vi "UHR-Fleezers Control (host) - 11.1.vi"() -> ()   [LabVIEW 2012] (continued)
                n290 = Multiply(x=w512, y=w521) -> (x*y=w531:dbl)
                n291 = Divide "X half step offset"(x=w509, y=2.0) -> (x/y=w517:dbl)
                n292 = Divide "X V/pix"(x=w509, y=w520) -> (x/y=w519:dbl)
                n293 = Multiply(x=w509, y=w514) -> (x*y=w526:dbl)
                n294 = Compound Arithmetic op=ADD(w524, w531, w530) -> (w501:dbl)
                "Pointer Y (V)" <- w501
                n295 = Multiply(x=w519, y=w513) -> (x*y=w528:dbl)
                n296 = Negate(x=w517) -> (-x=w516:dbl)
                n297 = local read "Initial X"() -> (w529:dbl)
                n298 = Negate(x=w528) -> (-x=w527:dbl)
                n299 = Compound Arithmetic op=ADD(w516, w526, w529, w527) -> (w502:dbl)
                "Pointer X (V)" <- w502
                n300 = case shown="True" "Set High F Confocal Spot (X-Y)" {
                  tunnel: w502 -> [_ w532]
                  tunnel: w501 -> [_ w533]
                  frame False {
                  }
                  frame True {
                    "Confocal Y 2 (V)" <- w533
                    "Confocal X 2 (V)" <- w532
                  }
                }
                n301 = Or(x="Set X Only", y="Set Confocal Spot (X-Y)") -> (x .or. y?=w505:bool)
                n302 = Or(x="Set Confocal Spot (X-Y)", y="Set Y Only") -> (x .or. y?=w504:bool)
                n303 = case shown="True" w505 {
                  tunnel: w502 -> [_ w534]
                  frame False {
                  }
                  frame True {
                    n304 = property on="AO2" class="Slide (strict)"("Val(Sgnl)"=w534) -> ()  [unwired: 2 in, 2 out]
                    "Confocal X 1 (V)" <- w534
                  }
                }
                n305 = case shown="True" w504 {
                  tunnel: w501 -> [_ w535]
                  frame False {
                  }
                  frame True {
                    n306 = property on="AO1" class="Slide (strict)"("Val(Sgnl)"=w535) -> ()  [unwired: 2 in, 2 out]
                    "Confocal Y 1 (V)" <- w535
                  }
                }
                n307 = local write "Set High F Confocal Spot (X-Y)"(w500) -> ()
                n308 = local write "Set Confocal Spot (X-Y)"(w500) -> ()
                n309 = local write "Set X Only"(w500) -> ()
                n310 = local write "Set Y Only"(w500) -> ()
              }
            }
          }
          frame 3 {
            n311 = local read "BD 2 Frequency 1 (MHz)"() -> (w536:dbl)
            n312 = local read "BD 1 Frequency 1 (MHz)"() -> (w537:dbl)
            n313 = local write "Manipulating Trap"(TRUE ("Manipulating Trap")) -> ()
            n314 = local write "Coords"(T7 {"Horizontal"=0, "Vertical"=0} ("Coords")) -> ()
            n315 = while {
              tunnel: w542 -> [w547]
              tunnel: w540 -> [w546]
              tunnel: w538 -> [w545]
              tunnel: w537 -> [w544]
              tunnel: w536 -> [w543]
              stop <- w548 stop-if-true
              n316 = event shown="[0] \"Pane\": Mouse Move" {
                selector: _ -> [_ _]
                dyn-events: _ -> [_ _]
                timeout: _ -> [_ _]
                tunnel: ["Force Manip Abort" w612] -> w548
                tunnel: w547 -> [w555 _]
                tunnel: w546 -> [w553 _]
                tunnel: w545 -> [w552 _]
                tunnel: w544 -> [w551 _]
                tunnel: w543 -> [w550 _]
                event Mouse Move {
                  n317 = event-data() -> ("Time"=w556:u32, "Coords"=w557:T7)  [unwired: 3 out]
                  n318 = Less?(x=w556, y=w555) -> (x < y?=w554:bool)
                  n319 = case "Makes sure old motion events prior to mouse click aren't used" shown="False" w554 {
                    tunnel: w557 -> [w599 _]
                    tunnel: w553 -> [w600 _]
                    tunnel: w552 -> [w577 _]
                    tunnel: w551 -> [w573 _]
                    tunnel: w550 -> [w572 _]
                    frame False {
                      n320 = Subtract(x=w599, y=w600) -> (x-y=w598:T7)
                      "Coords" <- w598
                      n321 = local read "Y RF Frequency Limits (MHz)"() -> (w558:T16)
                      n322 = To Double Precision Float(number=w598) -> (double precision float=w597:cluster{"Horizontal":dbl, "Vertical":dbl})
                      n323 = Multiply(x=cluster{"Horizontal":dbl, "Vertical":dbl} {"Horizontal"=-1.0, "Vertical"=1.0}, y="Manipulation Scaling") -> (x*y=w593:cluster{"Horizontal":dbl, "Vertical":dbl})
                      n324 = local read "X RF Frequency Limits (MHz)"() -> (w559:T16)
                      n325 = Multiply(x=w597, y=w593) -> (x*y=w595:cluster{"Horizontal":dbl, "Vertical":dbl})
                      n326 = Unbundle By Name(w595) -> ("Horizontal"=w590:dbl, "Vertical"=w594:dbl)
                      n327 = Unbundle By Name(w558) -> ("Maximum"=w561:dbl, "Minimum"=w560:dbl)
                      n328 = Boolean To (0,1)(Boolean="Manip. X?") -> (0, 1=w588:i16)
                      n329 = Boolean To (0,1)(Boolean="Manip. Y?") -> (0, 1=w585:i16)
                      n330 = local read "BD 1 Frequency 2 (MHz)"() -> (w575:dbl)
                      n331 = Multiply(x=w594, y=w585) -> (x*y=w587:dbl)
                      n332 = Multiply(x=w588, y=w590) -> (x*y=w591:dbl)
                      n333 = local read "BD 2 Frequency 2 (MHz)"() -> (w574:dbl)
                      n334 = Unbundle By Name(w559) -> ("Maximum"=w563:dbl, "Minimum"=w562:dbl)
                      n335 = Add(x=w572, y=w587) -> (x+y=w565:dbl)
                      n336 = Add(x=w573, y=w591) -> (x+y=w567:dbl)
                      n337 = In Range and Coerce(upper limit=w563, x=w567, lower limit=w562) -> (coerced(x)=w566:dbl)  [unwired: 1 out]
                      n338 = In Range and Coerce(upper limit=w561, x=w565, lower limit=w560) -> (coerced(x)=w564:dbl)  [unwired: 1 out]
                      n339 = Subtract(x=w566, y=w575) -> (x-y=w584:dbl)
                      n340 = Subtract(x=w564, y=w574) -> (x-y=w583:dbl)
                      n341 = Square(x=w584) -> (x^2=w582:dbl)
                      n342 = Square(x=w583) -> (x^2=w581:dbl)
                      n343 = Add(x=w582, y=w581) -> (x+y=w580:dbl)
                      n344 = Square Root(x=w580) -> (sqrt(x)=w576:dbl)
                      n345 = In Range and Coerce(upper limit="Limit Max (MHz)", x=w576, lower limit="Limit Min (MHz)") -> (In Range?=w569:bool)  [unwired: 1 out]
                      n346 = Not(x="Limits Enable") -> (.not. x?=w568:bool)
                      n347 = Or(x=w569, y=w568) -> (x .or. y?=w570:bool)
                      n348 = case shown="True" w570 {
                        tunnel: w577 -> [_ w610]
                        tunnel: w576 -> [_ w601]
                        tunnel: w566 -> [_ w608]
                        tunnel: w575 -> [_ w607]
                        tunnel: w564 -> [_ w606]
                        tunnel: w574 -> [_ w605]
                        tunnel: w559 -> [_ w603]
                        tunnel: w558 -> [_ w602]
                        frame False {
                        }
                        frame True {
                          n349 = local read "BD 1 Frequency 3 (MHz)"() -> (w609:dbl)
                          n350 = local read "BD 2 Frequency 3 (MHz)"() -> (w604:dbl)
                          n351 = local write "Trap Delta (MHz)"(w601) -> ()
                          n352 = call "set RF board frequency - interlace.vi"("Board 2 Frequency Limits"=w602, "Board 1 Frequency Limits"=w603, "FPGA VI Reference In"=w610, "Board 2 Frequency 3 (MHz)"=w604, "Board 1 Frequency 3 (MHz)"=w609, "Board 2 Frequency 2 (MHz)"=w605, "Board 2 Frequency 1 (MHz)"=w606, "Board 1 Frequency 2 (MHz)"=w607, "Board 1 Frequency 1  (MHz)"=w608) -> ()  [unwired: 1 in, 2 out]
                          n353 = local write "BD 2 Frequency 1 (MHz)"(w606) -> ()
                          n354 = local write "BD 1 Frequency 1 (MHz)"(w608) -> ()
                        }
                      }
                    }
                    frame True {
                    }
                  }
                }
                event Mouse Up {
                  n355 = event-data() -> ("Button"=w611:u16)  [unwired: 8 out]
                  n356 = case shown="3" w611 {
                    tunnel: [FALSE TRUE] -> w612
                    frame 0, Default {
                    }
                    frame 3 {
                      n357 = local read "Trap Delta (MHz)"() -> (w614:dbl)
                      n358 = property on="Initial delta (MHz)" class="DigNum (strict)"("Val(Sgnl)"=w614) -> ()  [unwired: 2 in, 2 out]
                      n359 = local write "Manipulating Trap"(FALSE ("Manipulating Trap")) -> ()
                    }
                  }
                }
              }
            }
          }
        }
      }
      event Mouse Move {
        n360 = event-data() -> ()  [unwired: 6 out]
      }
    }
    n361 = local read "Stop All"() -> (w430:bool)
    n362 = node-c288() -> ()  [unwired: 2 out]
  }
  n363 = timed-loop "Run Scripts, including: stage motion" {
    tunnel: w89 -> [w623]
    tunnel: w88 -> [w624]
    tunnel: [w624] -> w87
    tunnel: [w623] -> w86
    timing: w84 -> [_]
    timing-out: [_] -> w83
    tunnel: w69 -> [w622]
    tunnel: w70 -> [w621]
    tunnel: w10 -> [w618]
    tunnel: w9 -> [w617]
    tunnel: w8 -> [w619]
    tunnel: w7 -> [w620]
    stop <- w625 stop-if-true
    n364 = node-c288() -> ()  [unwired: 1 in, 1 out]
    n365 = event shown="[3] \"Move Cap. 2 (ADig Top)\": Value Change" {
      selector: _ -> [_ _ _ _ _ _ _ _ _ _ _ _ _ _ _ _ _ _ _]
      dyn-events: _ -> [_ _ _ _ _ _ _ _ _ _ _ _ _ _ _ _ _ _ _]
      timeout: _ -> [_ _ _ _ _ _ _ _ _ _ _ _ _ _ _ _ _ _ _]
      tunnel: ["Set Position" "Move to Position" _ _ "Read Harvard" _ _ _ _ _ _ "Got ADig bead" "Force FB Data\nScript" _ "Got DNA bead" "Take Stepping Data" _ "Take Detection Laser\nImage" _] -> _
      tunnel: [_ _ _ _ _ _ _ _ _ _ _ _ _ _ _ _ _ _ w1242] -> w625
      tunnel: w623 -> [w643 w651 w664 w694 _ w739 w779 w860 w889 w1021 w1047 _ w1083 _ _ _ _ _ _]
      tunnel: w624 -> [w644 w652 w665 w695 _ w740 w780 w861 w890 w1022 w1048 _ w1084 _ _ _ _ _ _]
      tunnel: w622 -> [_ _ _ _ w724 _ _ _ _ _ _ _ _ _ _ _ _ _ _]
      tunnel: w621 -> [_ _ _ _ w723 _ _ _ _ _ _ _ _ _ _ _ _ _ _]
      tunnel: w620 -> [_ _ _ _ _ _ _ _ _ _ _ _ _ _ _ _ _ _ _]
      tunnel: w619 -> [_ _ _ _ _ _ _ _ _ _ _ _ _ _ _ _ _ _ _]
      tunnel: w618 -> [_ _ _ _ _ _ _ _ _ _ _ _ _ _ _ _ _ _ _]
      tunnel: w617 -> [_ _ _ _ _ _ _ _ _ _ _ _ _ _ _ _ _ _ _]
      event "Set Position", "Set Position 2", "Set Position 3", "Set Position 4", "Set Position 5", "Set Position 1": Value Change {
        n366 = event-data() -> ()  [unwired: 1 in, 5 out]
        n367 = Build Array("Set Position 1", "Set Position 2", "Set Position 3", "Set Position 4", "Set Position 5") -> (w642:bool[])
        n368 = Boolean Array To Number(Boolean array=w642) -> (number=w641:u32)
        n369 = Logarithm Base 2(1:w641) -> (0:w633:dbl)
        n370 = call "Read Stage Position.vi"("error in"=w643, "VISA resource name in"=w644) -> ("Current Position"=w648:cluster{dbl, dbl, dbl}, "error out"=w647:errorcluster)  [unwired: 2 out]
        n371 = Decrement(x="Position") -> (x-1=w631:dbl)
        n372 = Greater Or Equal?(x=w633, y=0.0) -> (x >= y?=w634:bool)
        n373 = Cluster To Array(cluster=w648) -> (array=w645:dbl[])
        n374 = local write "Stage Control Serial Error"(w647) -> ()
        n375 = Select(t=w633, s=w634, f=w631) -> (s? t:f=w630:dbl)
        n376 = Increment(x=w630) -> (x+1=w629:dbl)
        n377 = Build Array (concatenate)(w629, w645) -> (w628:dbl[])
        n378 = Replace Array Subset(array="Saved Stage Positions", new element=w628, index (row)=w630) -> (w646:dbl[][])  [unwired: 1 in]
        n379 = local write "Saved Stage Positions"(w646) -> ()
      }
      event "Move to Position": Value Change {
        n380 = event-data() -> ()  [unwired: 1 in, 5 out]
        n381 = flat-sequence {
          tunnel: w652 -> [w656]
          tunnel: w651 -> [w655]
          frame #0 {
            n382 = local read "Saved Stage Positions"() -> (w658:dbl[][])
            n383 = local read "Position"() -> (w657:dbl)
            n384 = local write "Stage Moving"(TRUE ("Stage Moving")) -> ()
            n385 = call "move to saved stage position.vi"("error in"=w655, "Stage VISA resource name in"=w656, "Position"=w657, "Saved Stage Positions"=w658) -> ("error out"=w654:errorcluster)  [unwired: 1 out]
            n386 = local write "Stage Control Serial Error"(w654) -> ()
          }
          frame #1 {
            n387 = call <vilib>:"Beep.vi"() -> ()  [unwired: 3 in, 9 out]
            n388 = local write "Stage Moving"(FALSE ("Stage Moving")) -> ()
          }
        }
      }
      event "Move Cap. 1 (DNA Bottom)": Value Change {
        n389 = event-data() -> ()  [unwired: 1 in, 5 out]
        n390 = local write "Move Cap. 1 (DNA Bottom)"(FALSE ("Move Cap. 1 (DNA Right)")) -> ()
        n391 = flat-sequence {
          tunnel: w664 -> [w667]
          tunnel: w665 -> [w668]
          tunnel: [w668] -> w662
          tunnel: [w667] -> w661
          tunnel: w662 -> [w670]
          tunnel: w661 -> [w669]
          frame #0 {
            n392 = property on="Sample Channel\nFlow" class="Bool (strict)"("Val(Sgnl)"="Cap 1 Samp Flow ON") -> ()  [unwired: 2 in, 2 out]
          }
          frame #1 {
            n393 = local read "Saved Stage Positions"() -> (w680:dbl[][])
            n394 = local write "Stage Moving"(TRUE ("Stage Moving")) -> ()
            n395 = Array Subset(array=w680, index (row)=0 ("index"), length (row)=1 ("length"), index (col)=1 ("index"), length (col)=3 ("length")) -> (w677:dbl[][])
            n396 = Reshape Array(w677, 3 ("dimension size")) -> (w675:dbl[])
            n397 = Array To Cluster(array=w675) -> (cluster=w674:cluster{"[0]":dbl, "[1]":dbl, "[2]":dbl})
            n398 = call "Set Stage Position.vi"("Position"=w674, "error in"=w669, "VISA resource name in"=w670) -> ("error out"=w673:errorcluster)  [unwired: 2 out]
            n399 = local write "Stage Control Serial Error"(w673) -> ()
          }
          frame #2 {
            n400 = local write "Stage Moving"(FALSE ("Stage Moving")) -> ()
            n401 = case shown="True" "Cap 1 Flow ON" {
              frame False {
              }
              frame True {
                n402 = property on="Inject Pump 1" class="Bool (strict)"("Val(Sgnl)"=TRUE ("Value (Signaling)")) -> ()  [unwired: 2 in, 2 out]
              }
            }
            n403 = call <vilib>:"Beep.vi"() -> ()  [unwired: 3 in, 9 out]
          }
          frame #3 {
            n404 = property on="Sample Channel\nFlow" class="Bool (strict)"("Val(Sgnl)"=FALSE ("Value (Signaling)")) -> ()  [unwired: 2 in, 2 out]
            n405 = local read "Cap. 2 BD T1?\n(ADig T1, DNA T2)"() -> (w687:bool)
            n406 = case shown="True" w687 {
              tunnel: "Cap 1 T ON" -> [w689 w690]
              frame False {
                n407 = property on="Trap 1 (ON/OFF)" class="Bool (strict)"("Val(Sgnl)"=w689) -> ()  [unwired: 2 in, 2 out]
              }
              frame True {
                n408 = property on="Trap 2 (ON/OFF)" class="Bool (strict)"("Val(Sgnl)"=w690) -> ()  [unwired: 2 in, 2 out]
              }
            }
            n409 = property on="Got DNA bead" class="Bool"("Key Focus"=TRUE) -> ()  [unwired: 2 in, 2 out]
          }
        }
      }
      event "Move Cap. 2 (ADig Top)": Value Change {
        n410 = event-data() -> ()  [unwired: 1 in, 5 out]
        n411 = local write "Move Cap. 2 (ADig Top)"(FALSE ("Move Cap. 2 (ADig Left)")) -> ()
        n412 = flat-sequence {
          tunnel: w694 -> [w697]
          tunnel: w695 -> [w698]
          tunnel: [w698] -> w692
          tunnel: [w697] -> w691
          tunnel: w692 -> [w701]
          tunnel: w691 -> [w700]
          frame #0 {
            n413 = property on="Sample Channel\nFlow" class="Bool (strict)"("Val(Sgnl)"="Cap 2 Samp Flow ON") -> ()  [unwired: 2 in, 2 out]
          }
          frame #1 {
            w699 = FALSE ("Value (Signaling)")
            n414 = local read "Saved Stage Positions"() -> (w711:dbl[][])
            n415 = local write "Stage Moving"(TRUE ("Stage Moving")) -> ()
            n416 = Array Subset(array=w711, index (row)=1 ("index"), length (row)=1 ("length"), index (col)=1 ("index"), length (col)=3 ("length")) -> (w708:dbl[][])
            n417 = Reshape Array(w708, 3 ("dimension size")) -> (w706:dbl[])
            n418 = property on="Trap 1 (ON/OFF)" class="Bool (strict)"("Val(Sgnl)"=w699) -> ()  [unwired: 2 in, 2 out]
            n419 = property on="Trap 1 (ON/OFF)" class="Bool (strict)"("Val(Sgnl)"=w699) -> ()  [unwired: 2 in, 2 out]
            n420 = Array To Cluster(array=w706) -> (cluster=w705:cluster{"[0]":dbl, "[1]":dbl, "[2]":dbl})
            n421 = call "Set Stage Position.vi"("Position"=w705, "error in"=w700, "VISA resource name in"=w701) -> ("error out"=w704:errorcluster)  [unwired: 2 out]
            n422 = local write "Stage Control Serial Error"(w704) -> ()
          }
          frame #2 {
            n423 = local write "Stage Moving"(FALSE ("Stage Moving")) -> ()
            n424 = call <vilib>:"Beep.vi"() -> ()  [unwired: 3 in, 9 out]
            n425 = case shown="True" "Cap 2 Flow ON" {
              frame False {
              }
              frame True {
                n426 = property on="Inject Pump 3" class="Bool (strict)"("Val(Sgnl)"=TRUE ("Value (Signaling)")) -> ()  [unwired: 2 in, 2 out]
              }
            }
          }
          frame #3 {
            n427 = property on="Sample Channel\nFlow" class="Bool (strict)"("Val(Sgnl)"=FALSE ("Value (Signaling)")) -> ()  [unwired: 2 in, 2 out]
            n428 = case shown="False" "Cap. 2 BD T1?\n(ADig T1, DNA T2)" {
              tunnel: "Cap 2 T ON" -> [w720 w721]
              frame False {
                n429 = property on="Trap 2 (ON/OFF)" class="Bool (strict)"("Val(Sgnl)"=w720) -> ()  [unwired: 2 in, 2 out]
              }
              frame True {
                n430 = property on="Trap 1 (ON/OFF)" class="Bool (strict)"("Val(Sgnl)"=w721) -> ()  [unwired: 2 in, 2 out]
              }
            }
            n431 = property on="Got ADig bead" class="Bool"("Key Focus"=TRUE) -> ()  [unwired: 2 in, 2 out]
          }
        }
      }
      event "Read Harvard": Value Change {
        n432 = event-data() -> ()  [unwired: 1 in, 5 out]
        n433 = Concatenate Strings("write buffer", "\r") -> (w726:string)
        n434 = VISA Write(VISA resource name=w724, write buffer=w726, error in (no error)=w723) -> (VISA resource name out=w735:refnum<visa-resource-name>, error out=w734:errorcluster)  [unwired: 1 out]
        n435 = stacked-sequence {
          tunnel: [w738] -> w733
          tunnel: w735 -> [w738]
          tunnel: w734 -> [w737]
          tunnel: [w737] -> w728
          frame #0 {
            n436 = Wait (ms)(milliseconds to wait=50) -> ()  [unwired: 1 out]
          }
        }
        n437 = property class="Instr"(reference=w733, error in=w728) -> (reference out=w732:refnum<visa-resource-name>, error out=w730:errorcluster, "Serial Settings:Number of Bytes at Serial Port"=w731:u32)
        "Serial Settings:Number of Bytes at Serial Port" <- w731
        n438 = VISA Read(VISA resource name=w732, byte count=w731, error in (no error)=w730) -> (read buffer=w729:string)  [unwired: 3 out]
        "read buffer" <- w729
        n439 = Fract/Exp String To Number(string=w729) -> ()  [unwired: 5 out]
      }
      event "+z", "-z": Value Change {
        n440 = event-data() -> ()  [unwired: 1 in, 5 out]
        n441 = flat-sequence {
          tunnel: w739 -> [w761]
          tunnel: w740 -> [w741]
          frame #0 {
            n442 = call "Read Stage Position.vi"("error in"=w761, "VISA resource name in"=w741) -> ("Current Position"=w746:cluster{dbl, dbl, dbl}, "error out"=w759:errorcluster, "VISA resource name out"=w760:refnum<visa-resource-name>)  [unwired: 1 out]
            n443 = local read "Saved Stage Positions"() -> (w770:dbl[][])
            n444 = Divide(x="z nudge increment (um)", y=1000.0) -> (x/y=w758:dbl)
            n445 = Boolean To (0,1)(Boolean="+z") -> (0, 1=w750:i16)
            n446 = Boolean To (0,1)(Boolean="-z") -> (0, 1=w751:i16)
            n447 = Array Subset(array=w770, index (row)=1 ("index"), length (row)=1 ("length"), index (col)=1 ("index"), length (col)=3 ("length")) -> (w767:dbl[][])
            n448 = Multiply(x=w750, y=w758) -> (x*y=w754:dbl)
            n449 = Multiply(x=w751, y=w758) -> (x*y=w752:dbl)
            n450 = Unbundle(w746) -> (w744:dbl, w743:dbl, w747:dbl)
            n451 = Negate(x=w752) -> (-x=w753:dbl)
            n452 = Reshape Array(w767, 3 ("dimension size")) -> (w765:dbl[])
            n453 = Add(x=w754, y=w753) -> (x+y=w755:dbl)
            n454 = Array To Cluster(array=w765) -> ()  [unwired: 1 out]
            n455 = Add(x=w755, y=w747) -> (x+y=w745:dbl)
            n456 = Bundle(cluster=w746, w744, w743, w745) -> (w742:cluster{dbl, dbl, dbl})
            n457 = call "Set Stage Position.vi"("Position"=w742, "error in"=w759, "VISA resource name in"=w760) -> ("error out"=w764:errorcluster)  [unwired: 2 out]
            n458 = local write "Stage Moving"(TRUE ("Stage Moving")) -> ()
            n459 = local write "Stage Control Serial Error"(w764) -> ()
          }
          frame #1 {
            n460 = local write "Stage Moving"(FALSE ("Stage Moving")) -> ()
            n461 = call <vilib>:"Beep.vi"() -> ()  [unwired: 3 in, 9 out]
          }
        }
      }
      event "Cal/Data Acq. Spot": Value Change {
        n462 = event-data() -> ()  [unwired: 1 in, 5 out]
        n463 = flat-sequence {
          tunnel: w779 -> [w783]
          tunnel: w780 -> [w784]
          tunnel: [w784] -> w776
          tunnel: [w783] -> w775
          tunnel: w776 -> [w789]
          tunnel: w775 -> [w788]
          tunnel: ["Cal @ (MHz)"] -> w773
          tunnel: [w793] -> w777
          tunnel: w773 -> [w793]
          tunnel: w777 -> [w802]
          tunnel: ["W/ Offset 1"] -> w774
          tunnel: w777 -> [w823]
          tunnel: w774 -> [w821]
          frame #0 {
            n464 = property on="Sample Channel\nFlow" class="Bool (strict)"("Val(Sgnl)"="Daq spot flow on") -> ()  [unwired: 2 in, 2 out]
            n465 = Wait (ms)(milliseconds to wait=u32 250) -> ()  [unwired: 1 out]
          }
          frame #1 {
            n466 = local read "Saved Stage Positions"() -> (w786:dbl[][])
            n467 = property on="Trap Delta (MHz)" class="DigNum (strict)"("Val(Sgnl)"="Cal @ (MHz)") -> ()  [unwired: 2 in, 2 out]
            n468 = local write "Stage Moving"(TRUE ("Stage Moving")) -> ()
            n469 = call "move to saved stage position.vi"("error in"=w788, "Stage VISA resource name in"=w789, "Position"="Cal Stage Position", "Saved Stage Positions"=w786) -> ("error out"=w787:errorcluster)  [unwired: 1 out]
            n470 = local write "Stage Control Serial Error"(w787) -> ()
          }
          frame #2 {
            n471 = local write "Stage Moving"(FALSE ("Stage Moving")) -> ()
            n472 = property on="Sample Channel\nFlow" class="Bool (strict)"("Val(Sgnl)"="Flow ON during cal?") -> ()  [unwired: 2 in, 2 out]
            n473 = call <vilib>:"Beep.vi"() -> ()  [unwired: 3 in, 9 out]
          }
          frame #3 {
            n474 = Wait (ms)(milliseconds to wait=u32 1000) -> ()  [unwired: 1 out]
          }
          frame #4 {
            n475 = property on="Save Calibration" class="Bool (strict)"("Val(Sgnl)"=TRUE ("Value (Signaling)")) -> ()  [unwired: 2 in, 2 out]
          }
          frame #5 {
            n476 = Wait (ms)(milliseconds to wait=u32 2000) -> ()  [unwired: 1 out]
          }
          frame #6 {
            # "Check to see if \nsaving done"
            n477 = while {
              stop <- w798 stop-if-true
              n478 = local read "Saving..."() -> (w799:bool)
              n479 = Wait (ms)(milliseconds to wait=u32 100) -> ()  [unwired: 1 out]
              n480 = Not(x=w799) -> (.not. x?=w798:bool)
            }
          }
          frame #7 {
            n481 = case shown="True" "W/ Offset 1" {
              tunnel: w802 -> [_ w803]
              frame False {
              }
              frame True {
                n482 = stacked-sequence {
                  tunnel: w803 -> [_ _ _ _ _ _ _ w820]
                  frame #0 {
                    n483 = property on="Trap Delta (MHz)" class="DigNum (strict)"("Val(Sgnl)"="Offset 1 Start (MHz)") -> ()  [unwired: 2 in, 2 out]
                    n484 = Replace Array Subset(array=u32[] [0] ("Index Values"), new element="Offset 1 Set", index=0) -> (w804:u32[])
                    n485 = property on="Saved AOD Raster Scan Parameter Sets" class="Arr (strict)"("Index Values"=w804) -> ()  [unwired: 2 in, 2 out]
                  }
                  frame #1 {
                    n486 = Wait (ms)(milliseconds to wait=u32 200) -> ()  [unwired: 1 out]
                  }
                  frame #2 {
                    n487 = property on="Load parameters" class="Bool (strict)"("Val(Sgnl)"=TRUE ("Value (Signaling)")) -> ()  [unwired: 2 in, 2 out]
                  }
                  frame #3 {
                    n488 = Wait (ms)(milliseconds to wait=u32 200) -> ()  [unwired: 1 out]
                  }
                  frame #4 {
                    n489 = property on="Trap Raster Scan" class="Bool (strict)"("Val(Sgnl)"=TRUE ("Value (Signaling)")) -> ()  [unwired: 2 in, 2 out]
                  }
                  frame #5 {
                    n490 = Wait (ms)(milliseconds to wait=u32 2000) -> ()  [unwired: 1 out]
                  }
                  frame #6 {
                    n491 = while {
                      stop <- w817 stop-if-true
                      n492 = local read "Raster Scanning..."() -> (w819:bool)
                      n493 = local read "Saving..."() -> (w815:bool)
                      n494 = Wait (ms)(milliseconds to wait=u32 100) -> ()  [unwired: 1 out]
                      n495 = Not(x=w815) -> (.not. x?=w814:bool)
                      n496 = Not(x=w819) -> (.not. x?=w816:bool)
                      n497 = And(x=w816, y=w814) -> (x .and. y?=w817:bool)
                    }
                  }
                  frame #7 {
                    n498 = property on="Trap Delta (MHz)" class="DigNum (strict)"("Val(Sgnl)"=w820) -> ()  [unwired: 2 in, 2 out]
                  }
                }
              }
            }
          }
          frame #8 {
            n499 = local read "Save ave N"() -> (w822:dbl)
            n500 = case shown="False" "W/ Offset 2" {
              tunnel: w823 -> [_ w830]
              tunnel: w822 -> [_ w829]
              tunnel: w821 -> [w825 _]
              frame False {
                n501 = case shown="False" w825 {
                  frame False {
                    n502 = Multiply(x="Cal read wait (s)", y=u32 1000 ("milliseconds to wait")) -> (x*y=w827:u32)
                    n503 = Wait (ms)(milliseconds to wait=w827) -> ()  [unwired: 1 out]
                  }
                  frame True {
                  }
                }
              }
              frame True {
                n504 = stacked-sequence {
                  tunnel: w830 -> [_ _ _ _ _ _ _ _ _ w851 _ _]
                  tunnel: w829 -> [_ _ _ _ _ _ _ _ _ w849 _ _]
                  frame #0 {
                    n505 = property on="Save ave N" class="DigNum (strict)"("Val(Sgnl)"=1.0 ("Value (Signaling)")) -> ()  [unwired: 2 in, 2 out]
                  }
                  frame #1 {
                    n506 = Wait (ms)(milliseconds to wait=u32 500) -> ()  [unwired: 1 out]
                  }
                  frame #2 {
                    n507 = property on="Trap Delta (MHz)" class="DigNum (strict)"("Val(Sgnl)"="Offset 2 Start (MHz)") -> ()  [unwired: 2 in, 2 out]
                    n508 = Replace Array Subset(array=u32[] [0] ("Index Values"), new element="Offset 2 Set", index=0) -> (w835:u32[])
                    n509 = property on="Saved AOD Raster Scan Parameter Sets" class="Arr (strict)"("Index Values"=w835) -> ()  [unwired: 2 in, 2 out]
                  }
                  frame #3 {
                    n510 = Wait (ms)(milliseconds to wait=u32 500) -> ()  [unwired: 1 out]
                  }
                  frame #4 {
                    n511 = property on="Load parameters" class="Bool (strict)"("Val(Sgnl)"=TRUE ("Value (Signaling)")) -> ()  [unwired: 2 in, 2 out]
                  }
                  frame #5 {
                    n512 = Wait (ms)(milliseconds to wait=u32 500) -> ()  [unwired: 1 out]
                  }
                  frame #6 {
                    n513 = property on="Trap Raster Scan" class="Bool (strict)"("Val(Sgnl)"=TRUE ("Value (Signaling)")) -> ()  [unwired: 2 in, 2 out]
                  }
                  frame #7 {
                    n514 = Wait (ms)(milliseconds to wait=u32 2000) -> ()  [unwired: 1 out]
                  }
                  frame #8 {
                    n515 = while {
                      stop <- w844 stop-if-true
                      n516 = local read "Raster Scanning..."() -> (w847:bool)
                      n517 = local read "Saving..."() -> (w845:bool)
                      n518 = Wait (ms)(milliseconds to wait=u32 100) -> ()  [unwired: 1 out]
                      n519 = Not(x=w845) -> (.not. x?=w843:bool)
                      n520 = Not(x=w847) -> (.not. x?=w846:bool)
                      n521 = And(x=w846, y=w843) -> (x .and. y?=w844:bool)
                    }
                  }
                  frame #9 {
                    n522 = property on="Trap Delta (MHz)" class="DigNum (strict)"("Val(Sgnl)"=w851) -> ()  [unwired: 2 in, 2 out]
                    n523 = property on="Saved AOD Raster Scan Parameter Sets" class="Arr (strict)"("Index Values"=u32[] [0]) -> ()  [unwired: 2 in, 2 out]
                    n524 = property on="Save ave N" class="DigNum (strict)"("Val(Sgnl)"=w849) -> ()  [unwired: 2 in, 2 out]
                  }
                  frame #10 {
                    n525 = Wait (ms)(milliseconds to wait=u32 500) -> ()  [unwired: 1 out]
                  }
                  frame #11 {
                    n526 = property on="Load parameters" class="Bool (strict)"("Val(Sgnl)"=TRUE ("Value (Signaling)")) -> ()  [unwired: 2 in, 2 out]
                  }
                }
              }
            }
          }
          frame #9 {
            n527 = property on="Read Cal" class="Bool (strict)"("Val(Sgnl)"=TRUE ("Value (Signaling)")) -> ()  [unwired: 2 in, 2 out]
          }
          frame #10 {
            n528 = Wait (ms)(milliseconds to wait=u32 1000) -> ()  [unwired: 1 out]
          }
          frame #11 {
            n529 = property on="Fish for Tether" class="Bool (strict)"("Val(Sgnl)"=TRUE ("Value (Signaling)")) -> ()  [unwired: 2 in, 2 out]
          }
        }
        n530 = local write "Cal/Data Acq. Spot"(FALSE ("Cal/Data Acq. Spot")) -> ()
      }
      event "Dump Beads": Value Change {
        n531 = event-data() -> ()  [unwired: 1 in, 5 out]
        n532 = flat-sequence {
          tunnel: ["Dump spot flow on?"] -> w857
          tunnel: [w868] -> w858
          tunnel: w857 -> [w868]
          tunnel: w861 -> [w873]
          tunnel: w860 -> [w872]
          tunnel: [w870] -> w859
          tunnel: w858 -> [w870]
          tunnel: w859 -> [w883]
          frame #0 {
            w862 = FALSE ("Value (Signaling)")
            n533 = local read "Saving..."() -> (w864:bool)
            n534 = local write "Dump Beads"(FALSE ("Dump Beads")) -> ()
            n535 = property on="Inject Pump 3" class="Bool (strict)"("Val(Sgnl)"=w862) -> ()  [unwired: 2 in, 2 out]
            n536 = property on="Inject Pump 1" class="Bool (strict)"("Val(Sgnl)"=w862) -> ()  [unwired: 2 in, 2 out]
            n537 = local write "Stop Saving"(w864) -> ()
          }
          frame #1 {
            w865 = FALSE ("Fl. Triggered...")
            n538 = case shown="True" "Dump spot flow on?" {
              frame False {
              }
              frame True {
                n539 = property on="Sample Channel\nFlow" class="Bool (strict)"("Val(Sgnl)"=TRUE ("Stage Moving")) -> ()  [unwired: 2 in, 2 out]
              }
            }
            n540 = local write "Fl. Triggered..."(w865) -> ()
            n541 = local write "Tether"(w865) -> ()
            n542 = property on="Green Laser ON/Interlacing" class="Bool (strict)"("Val(Sgnl)"=w865) -> ()  [unwired: 2 in, 2 out]
            n543 = property on="Trap Pos. FB ON" class="Bool (strict)"("Val(Sgnl)"=w865) -> ()  [unwired: 2 in, 2 out]
            n544 = property on="Trap Trig. Fl." class="Bool (strict)"("Val(Sgnl)"=w865) -> ()  [unwired: 2 in, 2 out]
            n545 = property on="Fl. Triggered..." class="Bool (strict)"("Val(Sgnl)"=w865) -> ()  [unwired: 2 in, 2 out]
            n546 = property on="Dip for Protein" class="Bool (strict)"("Val(Sgnl)"=w865) -> ()  [unwired: 2 in, 2 out]
            n547 = property on="Pause dwell" class="Bool (strict)"("Val(Sgnl)"=w865) -> ()  [unwired: 2 in, 2 out]
          }
          frame #2 {
            n548 = property on="Trap Pos. FB Offset Factor" class="DigNum (strict)"("Val(Sgnl)"=i64 0 ("Value (Signaling)")) -> ()  [unwired: 2 in, 2 out]
          }
          frame #3 {
            n549 = local read "Saved Stage Positions"() -> (w874:dbl[][])
            n550 = local write "Stage Moving"(TRUE ("Stage Moving")) -> ()
            n551 = Array Subset(array=w874, index (row)=3 ("index"), length (row)=1 ("length"), index (col)=1 ("index"), length (col)=3 ("length")) -> (w879:dbl[][])
            n552 = Reshape Array(w879, 3 ("dimension size")) -> (w877:dbl[])
            n553 = Array To Cluster(array=w877) -> (cluster=w876:cluster{"[0]":dbl, "[1]":dbl, "[2]":dbl})
            n554 = call "Set Stage Position.vi"("Position"=w876, "error in"=w872, "VISA resource name in"=w873) -> ()  [unwired: 3 out]
          }
          frame #4 {
            w884 = FALSE ("Value (Signaling)")
            n555 = case shown="True" w883 {
              frame False {
              }
              frame True {
                n556 = property on="Sample Channel\nFlow" class="Bool (strict)"("Val(Sgnl)"=FALSE ("Stage Moving")) -> ()  [unwired: 2 in, 2 out]
              }
            }
            n557 = property on="Trap 1 (ON/OFF)" class="Bool (strict)"("Val(Sgnl)"=w884) -> ()  [unwired: 2 in, 2 out]
            n558 = property on="Trap 2 (ON/OFF)" class="Bool (strict)"("Val(Sgnl)"=w884) -> ()  [unwired: 2 in, 2 out]
            n559 = call <vilib>:"Beep.vi"() -> ()  [unwired: 3 in, 9 out]
          }
          frame #5 {
            n560 = property on="Move Cap. 2 (ADig Top)" class="Bool (strict)"("Val(Sgnl)"=TRUE ("Value (Signaling)")) -> ()  [unwired: 2 in, 2 out]
            n561 = property on="Tab Control" class="TabCtl (strict)"("Val(Sgnl)"=T4."Status" ("Value (Signaling)")) -> ()  [unwired: 2 in, 2 out]
          }
        }
      }
      event "Dip for Protein": Value Change {
        n562 = event-data() -> ()  [unwired: 1 in, 5 out]
        n563 = case shown="True" "Dip for Protein" {
          tunnel: w890 -> [_ w892]
          tunnel: w889 -> [_ w891]
          frame False {
          }
          frame True {
            n564 = while {
              tunnel: w892 -> [w903]
              tunnel: w891 -> [w902]
              i -> [w897]
              stop <- w899 stop-if-true
              n565 = Increment(x=w897) -> (x+1=→"Dip #":i32)
              n566 = flat-sequence {
                tunnel: w902 -> [w914]
                tunnel: w903 -> [w915]
                tunnel: [w915] -> w907
                tunnel: [w914] -> w906
                tunnel: [w908] -> w893
                tunnel: [w920] -> w901
                tunnel: [w921] -> w900
                tunnel: w907 -> [w922]
                tunnel: w906 -> [w923]
                tunnel: [w918] -> w894
                tunnel: w893 -> [w918]
                tunnel: [w931] -> w905
                tunnel: w901 -> [w931]
                tunnel: [w930] -> w904
                tunnel: w900 -> [w930]
                tunnel: [w927] -> w898
                tunnel: [w926] -> w895
                tunnel: w894 -> [w926]
                tunnel: w904 -> [w951]
                tunnel: w905 -> [w952]
                tunnel: w898 -> [w953]
                tunnel: w895 -> [w950]
                tunnel: [w1009] -> w899
                frame #0 {
                  n567 = local read "Trap Pos. FB ON"() -> (w908:bool)
                  n568 = Compound Arithmetic op=AND("Flow ON\nduring dip?", "FB OFF when \nflow ON", w908) -> (w909:bool)
                  n569 = case shown="True" "Move trap \nbefore dip move?" {
                    frame False {
                    }
                    frame True {
                      n570 = property on="Trap Delta (MHz)" class="DigNum (strict)"("Val(Sgnl)"="Dipping Delta (MHz)") -> ()  [unwired: 2 in, 2 out]
                    }
                  }
                  n571 = property on="Green Laser ON/Interlacing" class="Bool (strict)"("Val(Sgnl)"="Green ON\nbefore dip?") -> ()  [unwired: 2 in, 2 out]
                  n572 = property on="Sample Channel\nFlow" class="Bool (strict)"("Val(Sgnl)"="Flow ON\nduring dip?") -> ()  [unwired: 2 in, 2 out]
                  n573 = case shown="True" w909 {
                    frame False {
                    }
                    frame True {
                      n574 = property on="Trap Pos. FB ON" class="Bool (strict)"("Val(Sgnl)"=FALSE ("Value (Signaling)")) -> ()  [unwired: 2 in, 2 out]
                    }
                  }
                }
                frame #1 {
                  n575 = local read "Saved Stage Positions"() -> (w925:dbl[][])
                  n576 = local write "Cancel dwell"(FALSE ("Cancel dwell")) -> ()
                  n577 = call "move to saved stage position.vi"("error in"=w923, "Stage VISA resource name in"=w922, "Position"="Dip Stage \nPosition", "Saved Stage Positions"=w925) -> ("VISA resource name out"=w920:refnum<visa-resource-name>, "error out"=w921:errorcluster)
                }
                frame #2 {
                  n578 = node-c288() -> (w929:T21)  [unwired: 4 in]
                  n579 = timed-loop {
                    timing: w929 -> [_]
                    timing-out: [_] -> w928
                    tunnel: [w935] -> w927
                    i -> [w932]
                    stop <- w936 stop-if-true
                    n580 = node-c288() -> ()  [unwired: 1 in, 1 out]
                    n581 = Greater Or Equal?(x=w932, y="Dip Duration (s)") -> (x >= y?=w944:bool)
                    n582 = local read "Dip for Protein"() -> (w937:bool)
                    n583 = local read "Dump Beads"() -> (w934:bool)
                    n584 = local read "Cancel dwell"() -> (w943:bool)
                    n585 = local read "Pause dwell"() -> (w940:bool)
                    n586 = Not(x=w937) -> (.not. x?=w942:bool)
                    n587 = Compound Arithmetic op=OR(w943, w944, w942) -> (w941:bool)
                    n588 = Select(t=FALSE, s=w940, f=w941) -> (s? t:f=w938:bool)
                    n589 = Not(x=w934) -> (.not. x?=w933:bool)
                    n590 = node-c288() -> ()  [unwired: 1 in, 1 out]
                    n591 = And(x=w937, y=w933) -> (x .and. y?=w935:bool)
                    n592 = Or(x=w938, y=w934) -> (x .or. y?=w936:bool)
                    "Dip Time (s)" <- w932
                  }
                  n593 = node-c288(w928) -> ()  [unwired: 1 out]
                }
                frame #3 {
                  n594 = case shown="True" w953 {
                    tunnel: w952 -> [_ w958]
                    tunnel: w951 -> [_ w957]
                    tunnel: w950 -> [_ w954]
                    frame False {
                    }
                    frame True {
                      n595 = flat-sequence {
                        tunnel: w957 -> [w962]
                        tunnel: w958 -> [w963]
                        tunnel: [w963] -> w956
                        tunnel: [w962] -> w955
                        tunnel: w954 -> [w959]
                        tunnel: w956 -> [w973]
                        tunnel: w955 -> [w972]
                        tunnel: w954 -> [w981]
                        frame #0 {
                          n596 = local read "Sample Channel\nFlow"() -> (w961:bool)
                          n597 = case shown="True" w961 {
                            tunnel: "Flow ON \nduring return\nfrom dip?" -> [w964 w967]
                            tunnel: w959 -> [_ w966]
                            frame False {
                              n598 = case shown="True" w964 {
                                frame False {
                                }
                                frame True {
                                n599 = property on="Sample Channel\nFlow" class="Bool (strict)"("Val(Sgnl)"=TRUE ("Value (Signaling)")) -> ()  [unwired: 2 in, 2 out]
                                }
                              }
                            }
                            frame True {
                              n600 = case shown="False" w967 {
                                tunnel: w966 -> [w968 _]
                                frame False {
                                n601 = property on="Trap Pos. FB ON" class="Bool (strict)"("Val(Sgnl)"=w968) -> ()  [unwired: 2 in, 2 out]
                                n602 = property on="Sample Channel\nFlow" class="Bool (strict)"("Val(Sgnl)"=FALSE ("Value (Signaling)")) -> ()  [unwired: 2 in, 2 out]
                                }
                                frame True {
                                }
                              }
                            }
                          }
                        }
                        frame #1 {
                          # "For turning on green laser before stage reaches lower spot"
                          n603 = case shown="True" "Green ON\nafter start\nreturn?" {
                            frame False {
                            }
                            frame True {
                              n604 = flat-sequence {
                                frame #0 {
                                n605 = Multiply(x="Green delay after \nstart return (s)", y=1000.0) -> (x*y=w978:dbl)
                                n606 = Wait (ms)(milliseconds to wait=w978) -> ()  [unwired: 1 out]
                                }
                                frame #1 {
                                n607 = property on="Green Laser ON/Interlacing" class="Bool (strict)"("Val(Sgnl)"=TRUE ("Value (Signaling)")) -> ()  [unwired: 2 in, 2 out]
                                }
                              }
                            }
                          }
                          n608 = local read "Saved Stage Positions"() -> (w976:dbl[][])
                          n609 = local write "Cancel dwell"(FALSE ("Cancel dwell")) -> ()
                          n610 = call "move to saved stage position.vi"("error in"=w972, "Stage VISA resource name in"=w973, "Position"="Return Stage \nPosition", "Saved Stage Positions"=w976) -> ("error out"=w974:errorcluster)  [unwired: 1 out]
                          n611 = local write "Stage Control Serial Error"(w974) -> ()
                        }
                        frame #2 {
                          n612 = property on="Trap Pos. FB ON" class="Bool (strict)"("Val(Sgnl)"=w981) -> ()  [unwired: 2 in, 2 out]
                          n613 = case shown="True" "Green ON \nafter return?" {
                            frame False {
                            }
                            frame True {
                              n614 = property on="Green Laser ON/Interlacing" class="Bool (strict)"("Val(Sgnl)"=TRUE ("Value (Signaling)")) -> ()  [unwired: 2 in, 2 out]
                            }
                          }
                          n615 = case shown="True" "Move trap after return?" {
                            frame False {
                            }
                            frame True {
                              n616 = property on="Trap Delta (MHz)" class="DigNum (strict)"("Val(Sgnl)"="Dip Trap Delta 2 (MHz)") -> ()  [unwired: 2 in, 2 out]
                            }
                          }
                          n617 = case shown="True" "Save data after return?" {
                            frame False {
                            }
                            frame True {
                              n618 = property on="Start Saving" class="Bool (strict)"("Val(Sgnl)"=TRUE ("Value (Signaling)")) -> ()  [unwired: 2 in, 2 out]
                            }
                          }
                          n619 = property on="Sample Channel\nFlow" class="Bool (strict)"("Val(Sgnl)"="Flow ON\nduring daq?") -> ()  [unwired: 2 in, 2 out]
                        }
                        frame #3 {
                          n620 = node-c288() -> (w990:T21)  [unwired: 4 in]
                          n621 = timed-loop {
                            timing: w990 -> [_]
                            timing-out: [_] -> w989
                            i -> [w991]
                            stop <- w993 stop-if-true
                            n622 = node-c288() -> ()  [unwired: 1 in, 1 out]
                            n623 = local read "Dump Beads"() -> (w992:bool)
                            n624 = Greater Or Equal?(x=w991, y="Dwell Duration (s)") -> (x >= y?=w998:bool)
                            n625 = local read "Dip for Protein"() -> (w995:bool)
                            n626 = Not(x=w995) -> (.not. x?=w994:bool)
                            n627 = Compound Arithmetic op=OR(w998, "Cancel dwell", w994) -> (w997:bool)
                            n628 = node-c288() -> ()  [unwired: 1 in, 1 out]
                            n629 = Select(t=FALSE, s="Pause dwell", f=w997) -> (s? t:f=w1000:bool)
                            n630 = Or(x=w1000, y=w992) -> (x .or. y?=w993:bool)
                            "Dwell Time (s)" <- w991
                          }
                          n631 = node-c288(w989) -> ()  [unwired: 1 out]
                        }
                      }
                    }
                  }
                }
                frame #4 {
                  n632 = local read "Dip for Protein"() -> (w1010:bool)
                  n633 = local read "Dump Beads"() -> (w1007:bool)
                  n634 = local write "Cancel dwell"(FALSE ("Cancel dwell")) -> ()
                  n635 = Not(x=w1010) -> (.not. x?=w1011:bool)
                  n636 = Not(x="Cont. Repeat Dipping?") -> (.not. x?=w1013:bool)
                  n637 = Compound Arithmetic op=OR(w1011, w1013, w1007) -> (w1009:bool)
                }
              }
            }
          }
        }
      }
      event "Profile": Value Change {
        n638 = event-data() -> ()  [unwired: 1 in, 5 out]
        n639 = flat-sequence {
          tunnel: w1022 -> [w1025]
          tunnel: w1021 -> [w1033]
          tunnel: [w1027] -> w1020
          tunnel: [w1026] -> w1019
          tunnel: [w1024] -> w1017
          tunnel: [w1023] -> w1014
          tunnel: w1020 -> [w1040]
          tunnel: w1019 -> [w1039]
          tunnel: [w1037] -> w1018
          tunnel: w1017 -> [w1038]
          tunnel: [w1036] -> w1016
          tunnel: [w1035] -> w1015
          tunnel: w1014 -> [w1035]
          tunnel: w1018 -> [w1044]
          tunnel: w1016 -> [w1043]
          tunnel: w1015 -> [w1042]
          frame #0 {
            n640 = call "Read Stage Position.vi"("error in"=w1033, "VISA resource name in"=w1025) -> ("Current Position"=w1023:cluster{dbl, dbl, dbl}, "error out"=w1026:errorcluster, "VISA resource name out"=w1024:refnum<visa-resource-name>)  [unwired: 1 out]
            "Current Position" <- w1023
            n641 = local write "Stage Control Serial Error"(w1026) -> ()
            n642 = Unbundle(w1023) -> (w1030:dbl, w1032:dbl, w1028:dbl)
            n643 = Add(x=w1032, y="Y change (mm)") -> (x+y=w1029:dbl)
            n644 = Bundle(w1030, w1029, w1028) -> (w1027:cluster{dbl, dbl, dbl})  [unwired: 1 in]
          }
          frame #1 {
            # "move to new position and start saving"
            n645 = local write "Stage Moving"(TRUE ("Stage Moving")) -> ()
            n646 = local write "Start Saving"(TRUE ("Start Saving")) -> ()
            n647 = call "Set Stage Position.vi"("Position"=w1040, "error in"=w1039, "VISA resource name in"=w1038) -> ("error out"=w1036:errorcluster, "VISA resource name out"=w1037:refnum<visa-resource-name>)  [unwired: 1 out]
          }
          frame #2 {
            # "go back to start"
            n648 = call "Set Stage Position.vi"("Position"=w1042, "error in"=w1043, "VISA resource name in"=w1044) -> ()  [unwired: 3 out]
          }
          frame #3 {
            # "stop saving"
            n649 = local write "Stop Saving"(TRUE ("Stop Saving")) -> ()
            n650 = local write "Stage Moving"(FALSE ("Stage Moving")) -> ()
          }
        }
      }
      event "Move to Position 1", "Move to Position 2", "Move to Position 3", "Move to Position 4", "Move to Position 5", "Lower Ch. Cap.": Value Change {
        n651 = event-data() -> ()  [unwired: 1 in, 5 out]
        n652 = Or(x="Move to Position 5", y="Lower Ch. Cap.") -> (x .or. y?=w1050:bool)
        n653 = Build Array("Move to Position 1", "Move to Position 2", "Move to Position 3", "Move to Position 4", w1050) -> (w1053:bool[])
        n654 = Boolean Array To Number(Boolean array=w1053) -> (number=w1052:u32)
        n655 = Logarithm Base 2(1:w1052) -> (0:w1051:dbl)
        n656 = flat-sequence {
          tunnel: w1051 -> [w1062]
          tunnel: w1048 -> [w1060]
          tunnel: w1047 -> [w1059]
          frame #0 {
            n657 = local read "Saved Stage Positions"() -> (w1070:dbl[][])
            n658 = Array Subset(array=w1070, index (row)=w1062, length (row)=1 ("length"), index (col)=1 ("index"), length (col)=3 ("length")) -> (w1067:dbl[][])
            n659 = Reshape Array(w1067, 3 ("dimension size")) -> (w1065:dbl[])
            n660 = Array To Cluster(array=w1065) -> (cluster=w1064:cluster{"[0]":dbl, "[1]":dbl, "[2]":dbl})
            n661 = call "Set Stage Position.vi"("Position"=w1064, "error in"=w1059, "VISA resource name in"=w1060) -> ("error out"=w1063:errorcluster)  [unwired: 2 out]
            n662 = local write "Stage Moving"(TRUE ("Stage Moving")) -> ()
            n663 = local write "Stage Control Serial Error"(w1063) -> ()
          }
          frame #1 {
            n664 = local write "Stage Moving"(FALSE ("Stage Moving")) -> ()
            n665 = call <vilib>:"Beep.vi"() -> ()  [unwired: 3 in, 9 out]
          }
        }
      }
      event "Got ADig bead": Value Change {
        n666 = event-data() -> ()  [unwired: 1 in, 5 out]
        n667 = flat-sequence {
          frame #0 {
            n668 = local read "Cap 1 Samp Flow ON"() -> (w1074:bool)
            n669 = case shown="True" w1074 {
              frame False {
              }
              frame True {
                n670 = property on="Sample Channel\nFlow" class="Bool (strict)"("Val(Sgnl)"=TRUE ("Value (Signaling)")) -> ()  [unwired: 2 in, 2 out]
              }
            }
          }
          frame #1 {
            n671 = property on="Inject Pump 3" class="Bool (strict)"("Val(Sgnl)"=FALSE ("Value (Signaling)")) -> ()  [unwired: 2 in, 2 out]
          }
          frame #2 {
            n672 = property on="Move Cap. 1 (DNA Bottom)" class="Bool (strict)"("Val(Sgnl)"=TRUE ("Value (Signaling)")) -> ()  [unwired: 2 in, 2 out]
          }
        }
      }
      event "Force FB Data\nScript": Value Change {
        n673 = event-data() -> ()  [unwired: 1 in, 5 out]
        n674 = flat-sequence {
          tunnel: w1083 -> [w1087]
          tunnel: w1084 -> [w1088]
          tunnel: [w1088] -> w1079
          tunnel: [w1087] -> w1078
          tunnel: w1079 -> [w1091]
          tunnel: w1078 -> [w1090]
          tunnel: ["Trap Trig Fl."] -> w1080
          tunnel: [w1116] -> w1081
          tunnel: w1080 -> [w1116]
          tunnel: [w1120] -> w1082
          tunnel: w1081 -> [w1120]
          tunnel: w1082 -> [w1122]
          frame #0 {
            n675 = property on="Trap Delta (MHz)" class="DigNum (strict)"("Val(Sgnl)"="Trap Delta Before Moving") -> ()  [unwired: 2 in, 2 out]
          }
          frame #1 {
            n676 = local read "Saved Stage Positions"() -> (w1093:dbl[][])
            n677 = local write "FB Trap Pos Offset"(0.0 ("FB Trap Pos Offset")) -> ()
            n678 = property on="Trap Pos. FB Offset Factor" class="DigNum (strict)"("Val(Sgnl)"=i64 0 ("Value (Signaling)")) -> ()  [unwired: 2 in, 2 out]
            n679 = local write "Stage Moving"(TRUE ("Stage Moving")) -> ()
